vi "(PART 2) Exam Scores.vi"() -> ()   [LabVIEW 2018]
panel:
  out "Final Grade":dbl[](array[numeric])
  in  "Final Exam Scores":dbl[](array[numeric])
  in  "Exam 2 Scores":dbl[](array[numeric])
  in  "Exam 1 Scores":dbl[](array[numeric]) caption="Array"
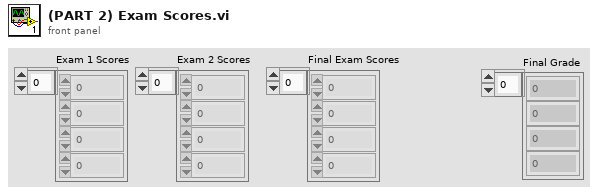
[diagram p1: front panel]
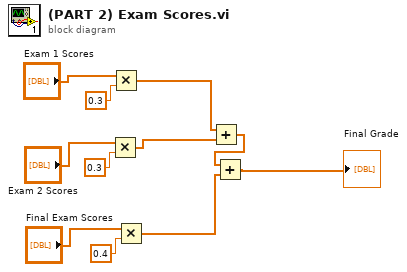
[diagram p0: block diagram]
diagram:
  n1 = Multiply(x="Exam 2 Scores", y=0.3) -> (x*y=w3:dbl[])
  n2 = Multiply(x="Exam 1 Scores", y=0.3) -> (x*y=w4:dbl[])
  n3 = Multiply(x="Final Exam Scores", y=0.4) -> (x*y=w2:dbl[])
  n4 = Add(x=w4, y=w3) -> (x+y=w11:dbl[])
  n5 = Add(x=w11, y=w2) -> (x+y=→"Final Grade":dbl[])
